vi "dfd_FXP PtByPt Cascaded SOS Form I Transposed.vi"(0 "x":T1={"value"=0, "wl"=0, "iwl"=0, "Signed"=TRUE} {"value" format="%.0x"}, 1 "coef b":i64[](array[numeric]), 2 "coef a":i64[](array[numeric]), 3 "#sec":i32, 5 "filtering statistics in":T4(array[cluster]) {"statistics information"."min value" format="%.2f"; "statistics information"."max value" format="%.2f"; "Quantizer Source" items=["Coefficients a/k"=0, "Coefficients b/v"=7, "Input"=1, "Output"=2, "Multiplicand"=3, "Product"=4, "Sum"=5, "Delay"=6]}, 6 "quantizers":T5[](array[typedef]) {"source" items=["Coef a/k"=0, "Coef b/v"=7, "Input"=1, "Output"=2, "Multiplicand"=3, "Product"=4, "Sum"=5, "Delay"=6, "Gain"=8]}, 7 "xState in":i64[](array[numeric]), 9 "yState in":i64[](array[numeric])) -> (11 "yState out":i64[](array[numeric]), 13 "xState out":i64[](array[numeric]), 14 "filtered x":T1={"value"=0, "wl"=0, "iwl"=0, "Signed"=TRUE} {"value" format="%.0x"}, 19 "filtering statistics out":T4(array[cluster]) {"statistics information"."min value" format="%.2f"; "statistics information"."max value" format="%.2f"; "Quantizer Source" items=["Coefficients a/k"=0, "Coefficients b/v"=7, "Input"=1, "Output"=2, "Multiplicand"=3, "Product"=4, "Sum"=5, "Delay"=6]})   [LabVIEW 2017, in "NI_DigFilter_FXP.lvlib"]
uses:
  <vilib>/addons/Digital Filter Design/NI_DigFilter_FXP.lvlib
  <vilib>/addons/Digital Filter Design/_Objects.llb/dfd_DFXP Data Type (scaler).ctl
  <vilib>/addons/Digital Filter Design/_Objects.llb/dfd_DFXP Operation Parameter.ctl
  <vilib>/addons/Digital Filter Design/_Objects.llb/dfd_Internal Quantization Srcs.ctl
  <vilib>/addons/Digital Filter Design/_Objects.llb/DFD Quantization Sources.ctl
  <vilib>/addons/Digital Filter Design/_Objects.llb/DFD FXP Statistics Data.ctl
  <vilib>/addons/Digital Filter Design/NI_DigFilterLicensed.lvlib
panel:
  in  "coef_b":T1={"value"=0, "wl"=0, "iwl"=0, "Signed"=TRUE} {"value" format="%.0x"}
  in  "coef_a":T1={"value"=0, "wl"=0, "iwl"=0, "Signed"=TRUE} {"value" format="%.0x"}
  in  "State":T1={"value"=0, "wl"=0, "iwl"=0, "Signed"=TRUE} {"value" format="%.0x"}
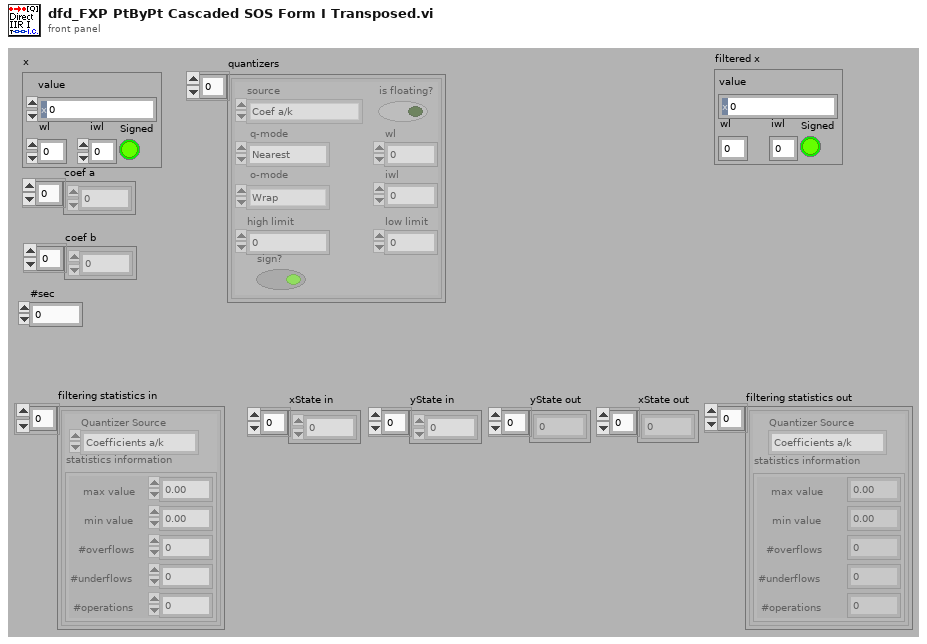
[diagram p1: front panel]
types:
  T1 = typedef "dfd_DFXP Data Type (scaler).ctl" = cluster{"value":i64, "wl":i16, "iwl":i16, "Signed":bool}
  T2 = typedef "NI_DigFilterLicensed.lvlib/DFD Quantization Sources.ctl" = u16
  T3 = typedef "NI_DigFilterLicensed.lvlib/DFD FXP Statistics Data.ctl" = cluster{"max value":ext, "min value":ext, "#overflows":i32, "#underflows":i32, "#operations":i32}
  T4 = cluster{"Quantizer Source":T2, "statistics information":T3}[]
  T5 = typedef "dfd_DFXP Operation Parameter.ctl" = cluster{"source":T6, "is floating?":bool, "o-mode":enum16{"Saturation", "Wrap"}, "q-mode":enum16{"Nearest", "Truncation"}, "wl":i16, "high limit":i64, "low limit":i64, "iwl":i16, "sign?":bool}
  T6 = typedef "NI_DigFilterLicensed.lvlib/dfd_Internal Quantization Srcs.ctl" = u16
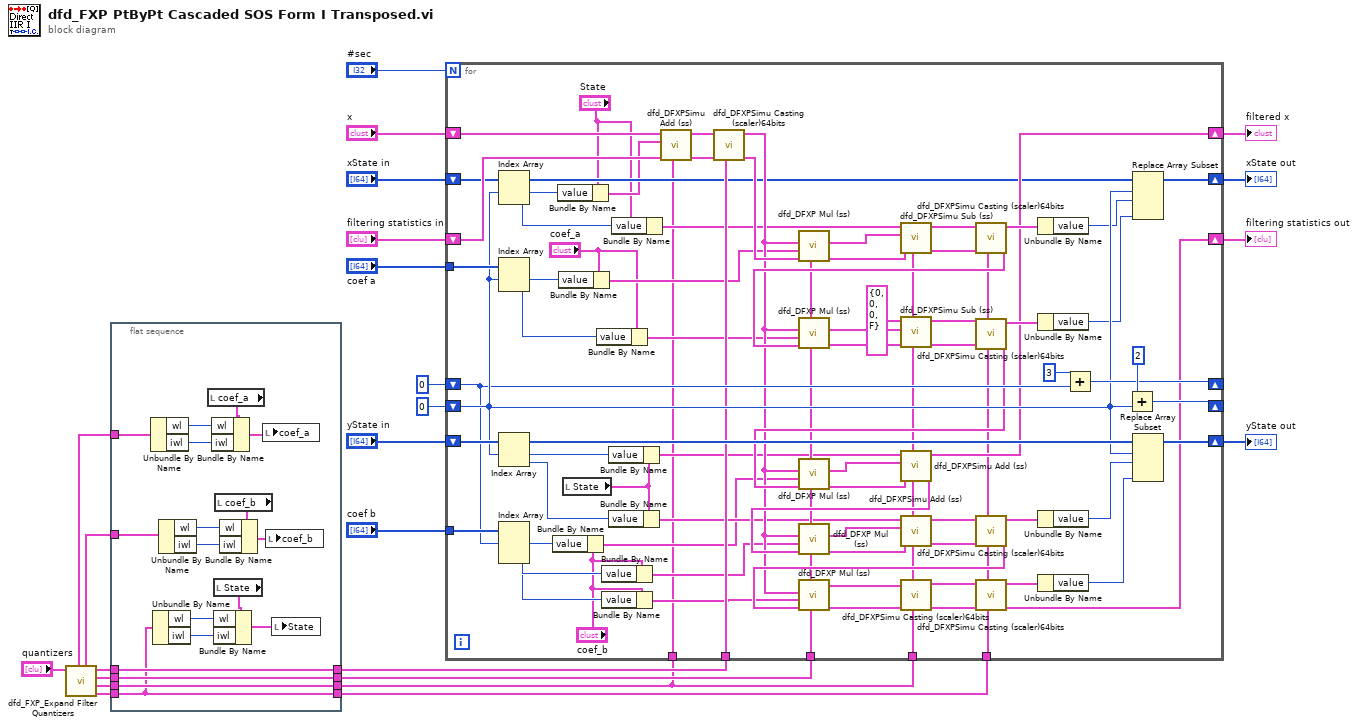
[diagram p0: block diagram]
diagram:
  n1 = call <vilib>:"dfd_FXP_Expand Filter Quantizers.vi"("FXPOPs"="quantizers") -> ("Delay"=w10:T5, "Sum"=w5:T5, "Product"=w7:T5, "Multiplicand"=w9:T5, "Coefficient b/v"=w3:T5, "Coefficient a/k"=w2:T5)  [unwired: 5 out]
  n2 = flat-sequence {
    tunnel: w10 -> [w35]
    tunnel: w9 -> [w38]
    tunnel: [w38] -> w8
    tunnel: [w37] -> w6
    tunnel: w7 -> [w37]
    tunnel: w5 -> [w36]
    tunnel: [w36] -> w1
    tunnel: [w35] -> w4
    tunnel: w3 -> [w33]
    tunnel: w2 -> [w27]
    frame #0 {
      n3 = Unbundle By Name(w27) -> ("wl"=w29:i16, "iwl"=w28:i16)
      n4 = Unbundle By Name(w35) -> ("wl"=w41:i16, "iwl"=w40:i16)
      n5 = Unbundle By Name(w33) -> ("wl"=w30:i16, "iwl"=w34:i16)
      n6 = local read "coef_a"() -> (w25:T1)
      n7 = Bundle By Name(cluster=w25, "wl"=w29, "iwl"=w28) -> (w26:T1)
      n8 = local read "State"() -> (w42:T1)
      n9 = Bundle By Name(cluster=w42, "wl"=w41, "iwl"=w40) -> (w39:T1)
      n10 = local read "coef_b"() -> (w31:T1)
      n11 = Bundle By Name(cluster=w31, "wl"=w30, "iwl"=w34) -> (w32:T1)
      n12 = local write "coef_a"(w26) -> ()
      n13 = local write "coef_b"(w32) -> ()
      n14 = local write "State"(w39) -> ()
    }
  }
  n15 = for {
    N: "#sec" -> [_]
    shift-right: [w118] -> w21
    shift-left: "yState in" -> [w119]
    shift-right: [w120] -> w23
    shift-left: "xState in" -> [w67]
    shift-right: [w117] -> _
    shift-left: 0 -> [w111]
    shift-right: [w100] -> w15
    shift-left: "x" -> [w109]
    shift-right: [w114] -> _
    shift-left: 0 -> [w110]
    tunnel: "coef a" -> [w113]
    tunnel: "coef b" -> [w112]
    tunnel: w8 -> [w80]
    tunnel: w6 -> [w79]
    tunnel: w1 -> [w48]
    tunnel: w4 -> [w78]
    tunnel: w1 -> [w49]
    shift-right: [w90] -> w11
    shift-left: "filtering statistics in" -> [w93]
    n16 = Index Array(array=w67, index #1=w111) -> (element #1=w108:i64, element #2=w106:i64)  [unwired: 1 in]
    n17 = Index Array(array=w113, index #1=w111) -> (element #1=w73:i64, element #2=w72:i64)  [unwired: 1 in]
    n18 = Index Array(array=w119, index #1=w111) -> (element #1=w101:i64, element #2=w97:i64)  [unwired: 1 in]
    n19 = Index Array(array=w112, index #1=w110) -> (element #1=w71:i64, element #2=w70:i64, element #3=w68:i64)  [unwired: 2 in]
    n20 = Bundle By Name(cluster="coef_b", "value"=w71) -> (w57:T1)
    n21 = Bundle By Name(cluster="State", "value"=w108) -> (w66:T1)
    n22 = Bundle By Name(cluster="coef_a", "value"=w73) -> (w63:T1)
    n23 = local read "State"() -> (w58:T1)
    n24 = Bundle By Name(cluster="coef_a", "value"=w72) -> (w62:T1)
    n25 = Bundle By Name(cluster="coef_b", "value"=w70) -> (w55:T1)
    n26 = Bundle By Name(cluster="coef_b", "value"=w68) -> (w56:T1)
    n27 = Bundle By Name(cluster=w58, "value"=w101) -> (w60:T1)
    n28 = Bundle By Name(cluster=w58, "value"=w97) -> (w59:T1)
    n29 = Bundle By Name(cluster="State", "value"=w106) -> (w65:T1)
    n30 = call <vilib>:"dfd_DFXPSimu Add (ss).vi"("op params"=w49, "filtering statistics in"=w93, "value in 2"=w66, "value in 1"=w109) -> ("filtering statistics out"=w92:T4, "value out"=w107:T1)  [unwired: 1 in, 5 out]
    n31 = call <vilib>:"dfd_DFXPSimu Casting (scaler)64bits.vi"("op params"=w80, "filtering statistics in"=w92, "Value in"=w107) -> ("filtering statistics out"=w91:T4, "Value out"=w69:T1)  [unwired: 2 in, 5 out]
    n32 = call <vilib>:"dfd_DFXP Mul (ss).vi"("op params"=w79, "filtering statistics in"=w91, "Value in 2"=w63, "Value in"=w69) -> ("filtering statistics out"=w89:T4, "Value out"=w103:T1)  [unwired: 6 out]
    n33 = call <vilib>:"dfd_DFXPSimu Sub (ss).vi"("op params"=w48, "filtering statistics in"=w89, "value in 2"=w103, "value in 1"=w65) -> ("filtering statistics out"=w88:T4, "value out"=w105:T1)  [unwired: 6 out]
    n34 = call <vilib>:"dfd_DFXPSimu Casting (scaler)64bits.vi"("op params"=w78, "filtering statistics in"=w88, "Value in"=w105) -> ("filtering statistics out"=w87:T4, "Value out"=w104:T1)  [unwired: 1 in, 6 out]
    n35 = call <vilib>:"dfd_DFXP Mul (ss).vi"("op params"=w79, "filtering statistics in"=w87, "Value in 2"=w62, "Value in"=w69) -> ("filtering statistics out"=w47:T4, "Value out"=w46:T1)  [unwired: 6 out]
    n36 = call <vilib>:"dfd_DFXPSimu Sub (ss).vi"("op params"=w48, "filtering statistics in"=w47, "value in 2"=w46, "value in 1"=T1 {"value"=0, "wl"=0, "iwl"=0, "Signed"=FALSE}) -> ("filtering statistics out"=w43:T4, "value out"=w44:T1)  [unwired: 6 out]
    n37 = call <vilib>:"dfd_DFXPSimu Casting (scaler)64bits.vi"("op params"=w78, "filtering statistics in"=w43, "Value in"=w44) -> ("filtering statistics out"=w86:T4, "Value out"=w102:T1)  [unwired: 1 in, 6 out]
    n38 = call <vilib>:"dfd_DFXP Mul (ss).vi"("op params"=w79, "filtering statistics in"=w86, "Value in 2"=w57, "Value in"=w69) -> ("filtering statistics out"=w85:T4, "Value out"=w99:T1)  [unwired: 6 out]
    n39 = call <vilib>:"dfd_DFXPSimu Add (ss).vi"("op params"=w48, "filtering statistics in"=w85, "value in 2"=w99, "value in 1"=w60) -> ("filtering statistics out"=w84:T4, "value out"=w100:T1)  [unwired: 6 out]
    n40 = call <vilib>:"dfd_DFXP Mul (ss).vi"("op params"=w79, "filtering statistics in"=w84, "Value in 2"=w55, "Value in"=w69) -> ("filtering statistics out"=w83:T4, "Value out"=w98:T1)  [unwired: 6 out]
    n41 = call <vilib>:"dfd_DFXPSimu Add (ss).vi"("op params"=w48, "filtering statistics in"=w83, "value in 2"=w98, "value in 1"=w59) -> ("filtering statistics out"=w82:T4, "value out"=w96:T1)  [unwired: 6 out]
    n42 = call <vilib>:"dfd_DFXPSimu Casting (scaler)64bits.vi"("op params"=w78, "filtering statistics in"=w82, "Value in"=w96) -> ("filtering statistics out"=w81:T4, "Value out"=w95:T1)  [unwired: 1 in, 6 out]
    n43 = call <vilib>:"dfd_DFXP Mul (ss).vi"("op params"=w79, "filtering statistics in"=w81, "Value in 2"=w56, "Value in"=w69) -> ("filtering statistics out"=w75:T4, "Value out"=w77:T1)  [unwired: 6 out]
    n44 = call <vilib>:"dfd_DFXPSimu Casting (scaler)64bits.vi"("op params"=w48, "filtering statistics in"=w75, "Value in"=w77) -> ("filtering statistics out"=w74:T4, "Value out"=w76:T1)  [unwired: 1 in, 6 out]
    n45 = call <vilib>:"dfd_DFXPSimu Casting (scaler)64bits.vi"("op params"=w78, "filtering statistics in"=w74, "Value in"=w76) -> ("filtering statistics out"=w90:T4, "Value out"=w94:T1)  [unwired: 1 in, 6 out]
    n46 = Unbundle By Name(w104) -> ("value"=w50:i64)
    n47 = Unbundle By Name(w102) -> ("value"=w51:i64)
    n48 = Unbundle By Name(w95) -> ("value"=w53:i64)
    n49 = Unbundle By Name(w94) -> ("value"=w52:i64)
    n50 = Add(x=3, y=w110) -> (x+y=w114:i32)
    n51 = Add(x=2 ("y"), y=w111) -> (x+y=w117:i32)
    n52 = Replace Array Subset(array=w67, new element #1=w50, index #1=w111, new element #2=w51) -> (w120:i64[])  [unwired: 1 in]
    n53 = Replace Array Subset(array=w119, new element #1=w53, index #1=w111, new element #2=w52) -> (w118:i64[])  [unwired: 1 in]
  }
  "filtered x" <- w15
  "xState out" <- w23
  "yState out" <- w21
  "filtering statistics out" <- w11
